vi "TestDLL.vi"() -> ()   [LabVIEW 2013]
uses:
  subvi/OpencvLabviewTest.lvlib
  subvi/OpencvLabviewTest.dll
panel:
  out "blured image":T1(plugin-control)
  in  "input height":dbl
  in  "input width":dbl
  out "show blank image":T1(plugin-control)
  out "original height":i32
  out "original width":i32
  out "image area":u32
  out "original image":T1(plugin-control)
  out "area":u32
  in  "width":u32
  in  "height":u32
  # "__declspec(dllexport) int area(int width, int height);"
  # "__declspec(dllexport) int area_from_image(IMAP_Image *imageSrc);"
  # "__declspec(dllexport) int show_blank_image(IMAP_Image *imageDst, int width, int height);"
  # "__declspec(dllexport) int image_blur(IMAP_Image *imageSrc, IMAP_Image *imageDst);"
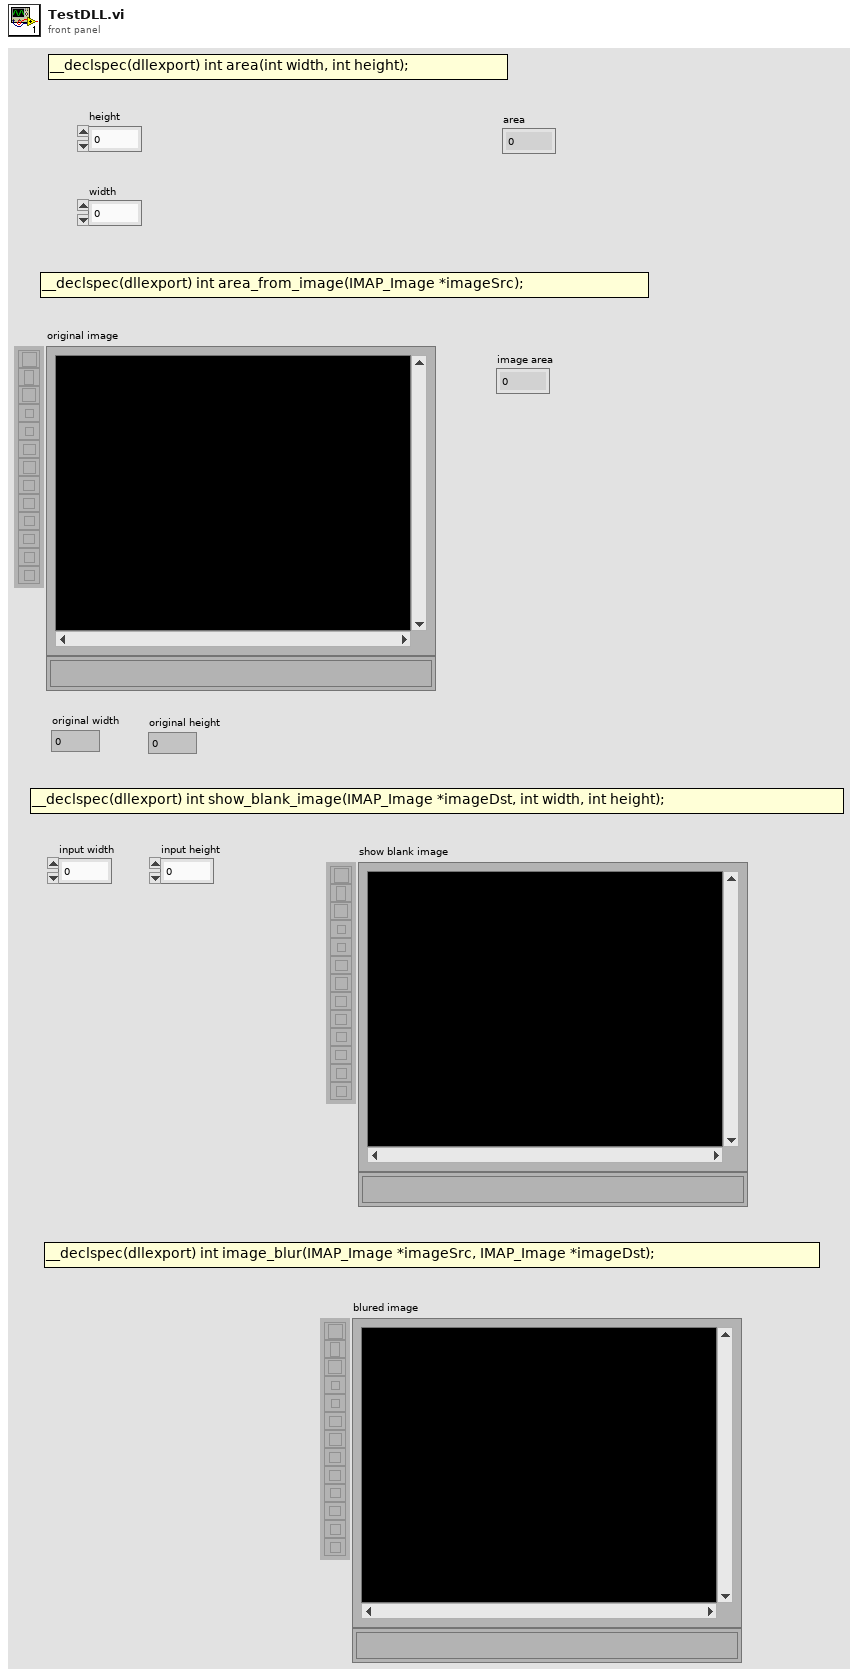
[diagram p1: front panel]
types:
  T1 = typedef "IMAQ Image.ctl" = refnum<image>
  T2 = typedef "Image Type" = u32
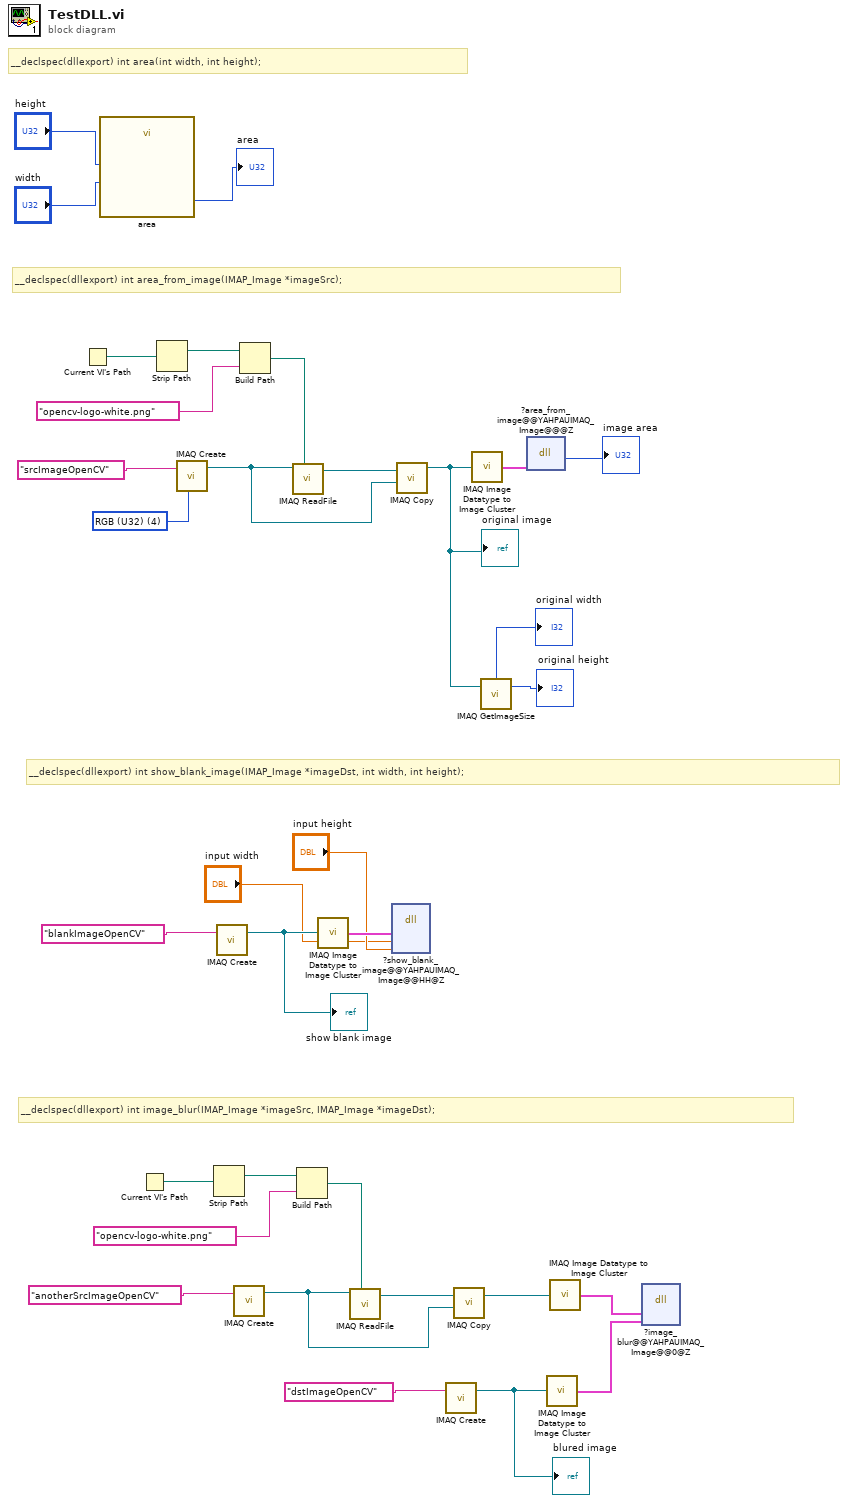
[diagram p0: block diagram]
diagram:
  w1 = T2 4 items=["Grayscale (U8)", "Grayscale (I16)", "Grayscale (SGL)", "Complex (CSG)", "RGB (U32)", "HSL (U32)", "RGB (U64)", "Grayscale (U16)"] ("Image Type")
  # "__declspec(dllexport) int image_blur(IMAP_Image *imageSrc, IMAP_Image *imageDst);"
  # "__declspec(dllexport) int show_blank_image(IMAP_Image *imageDst, int width, int height);"
  # "__declspec(dllexport) int area_from_image(IMAP_Image *imageSrc);"
  # "__declspec(dllexport) int area(int width, int height);"
  n1 = Current VI's Path() -> (path=w29:path)
  n2 = call "area.vi"("height"="height", "width"="width") -> ("function return"=→"area":i32)  [unwired: 9 in]
  n3 = Current VI's Path() -> (path=w9:path)
  n4 = Strip Path(path=w29) -> (stripped path=w28:path)  [unwired: 1 out]
  n5 = call "IMAQ Create"("Image Name"="srcImageOpenCV", "Image Type"=w1) -> ("New Image"=w20:T1)  [unwired: 3 in, 1 out]
  n6 = Strip Path(path=w9) -> (stripped path=w8:path)  [unwired: 1 out]
  n7 = call "IMAQ Create"("Image Name"="blankImageOpenCV") -> ("New Image"=w16:T1)  [unwired: 4 in, 1 out]
  "show blank image" <- w16
  n8 = call "IMAQ Create"("Image Name"="anotherSrcImageOpenCV") -> ("New Image"=w4:T1)  [unwired: 4 in, 1 out]
  n9 = Build Path(base path=w28, name or relative path="opencv-logo-white.png") -> (appended path=w27:path)
  n10 = call "IMAQ ReadFile"("File Path"=w27, "Image"=w20) -> ("Image Out"=w21:T1)  [unwired: 5 in, 4 out]
  n11 = Build Path(base path=w8, name or relative path="opencv-logo-white.png") -> (appended path=w7:path)
  n12 = call <vilib>:"IMAQ Image Datatype to Image Cluster.vi"("Image"=w16) -> ("Image (dup)"=w17:cluster{string, u32})
  n13 = call "IMAQ ReadFile"("File Path"=w7, "Image"=w4) -> ("Image Out"=w5:T1)  [unwired: 5 in, 4 out]
  n14 = dll-call lib="D:/congxin/Connectors/OpenCV-LabVIEW/LabVIEW/subvi/OpencvLabviewTest.dll" fn="?show_blank_image@@YAHPAUIMAQ_Image@@HH@Z"("imageDst"=w17, "width"="input width", "height"="input height") -> ()  [unwired: 7 in, 2 out]
  n15 = call "IMAQ Copy"("Image Dst"=w20, "Image Src"=w21) -> ("Image Dst Out"=w19:T1)  [unwired: 4 in, 1 out]
  "original image" <- w19
  n16 = call "IMAQ Create"("Image Name"="dstImageOpenCV") -> ("New Image"=w11:T1)  [unwired: 4 in, 1 out]
  "blured image" <- w11
  n17 = call "IMAQ Copy"("Image Dst"=w4, "Image Src"=w5) -> ("Image Dst Out"=w3:T1)  [unwired: 4 in, 1 out]
  n18 = call <vilib>:"IMAQ Image Datatype to Image Cluster.vi"("Image"=w19) -> ("Image (dup)"=w25:cluster{string, u32})
  n19 = call "IMAQ GetImageSize"("Image"=w19) -> ("Y Resolution"=→"original height":i32, "X Resolution"=→"original width":i32)  [unwired: 3 in, 1 out]
  n20 = dll-call lib="D:/congxin/Connectors/OpenCV-LabVIEW/LabVIEW/subvi/OpencvLabviewTest.dll" fn="?area_from_image@@YAHPAUIMAQ_Image@@@Z"("imageSrc"=w25) -> ("return type"=→"image area":u32)  [unwired: 4 in, 2 out]
  n21 = call <vilib>:"IMAQ Image Datatype to Image Cluster.vi"("Image"=w11) -> ("Image (dup)"=w12:cluster{string, u32})
  n22 = call <vilib>:"IMAQ Image Datatype to Image Cluster.vi"("Image"=w3) -> ("Image (dup)"=w2:cluster{string, u32})
  n23 = dll-call lib="D:/congxin/Connectors/OpenCV-LabVIEW/LabVIEW/subvi/OpencvLabviewTest.dll" fn="?image_blur@@YAHPAUIMAQ_Image@@0@Z"("imageSrc"=w2, "imageDst"=w12) -> ()  [unwired: 6 in, 2 out]
